vi "Main.vi"(8 "error in (no error)":errorcluster) -> (0 "error out":errorcluster)   [LabVIEW 2013]
doc: "Use this template to build a VI to use as a subVI."
uses:
  Instrument Module Typedefs/InstrumentStateEnum.ctl
  General TypeDefs/MeasurementType.ctl
  Instrument Module Typedefs/AbsorptionStateEnum.ctl
  General TypeDefs/FileSaveControllerEnum.ctl
  Measurement Typedefs/KineticNotifierDatatype.ctl
  Measurement Typedefs/MeasurementGFV.ctl
  General TypeDefs/ConfigurationDataTypeDef.ctl
  <vilib>/Utility/config.llb/Read Key (Double).vi
  <vilib>/Utility/config.llb/Read Key (Path).vi
  <vilib>/Utility/config.llb/Read Key (String).vi
  <vilib>/Utility/config.llb/Write Key (Path).vi
  <vilib>/Utility/config.llb/Write Key (String).vi
  <vilib>/Utility/config.llb/Write Key (Double).vi
  <instrlib>/Ocean Optics 2000 4000/Ocean Optics 2000 4000.lvlib
  <vilib>/Utility/config.llb/NI_LVConfig.lvlib
panel:
  in  "Export to Excel":bool
  in  "Open DB Button":bool
  in  "Save DB Button":bool
  out "Selected Wavelengths":dbl[](array[numeric])
  out "Read Status":string
  in  "Sample Name":string
  in  "MeasurementTabControl":T1(tab)=enum."Kinetic Measurement"
  out "Absorption Saved Results":T2(graph)
  out "Absorption @ wavelengths vs Time":T2(graph)
  out "Absorption Saved Results":T2(graph)
  out "Time to\nNext Save (s)":dbl=0.9000897407531738 caption="Elapsed Time (s)" format="%#.0f s"
  out "Save No.":i32
  out "FileSaveStateStatus":string="Stop" caption="File Recorder State"
  in  "Add Wavelength":bool
  in  "Remove Wavelength":bool
  in  "Measurement Type":T3=enum."Kinetic"
  in  "Req. No. of Saves":i32=1 min=1 max=10000 step=1
  in  "Enable\nAutomatic\nStop":bool=TRUE
  in  "Pause":bool caption="Start Cooling/Heating"
  in  "Stop Saves":bool caption="Start Cooling/Heating"
  in  "Record":bool caption="Start Cooling/Heating"
  in  "Time Between Consecutive Frames (sec)":dbl=1.0 caption="Time Between \nConsecutive \nSaves (sec)" min=0.0 max=3600.0 step=0.1 format="%.1f s"
  in  "Remarks":string
  out "Goal":string
  out "Experiment Name":string="tes"
  in  "NewExperiment":bool
  out "File Path":path=path "E:/LINKAM Measurements_Naama/20140915"
  in  "stop":bool
  in  "error in (no error) 2":errorcluster
  in  "Measurement Control":T4(tab)=enum."Setup Absorption Measurement"
  out "Selected Spectrometer":refnum<visa-resource-name>="USB650"
  in  "Save Calibration":bool
  out "Current State":T5=enum."Continuous Measurement"
  in  "Configure":bool
  in  "Continuous Measurement":bool
  in  "Stop Measurements":bool
  in  "Delay between measurements (ms)":i32=10 min=10 max=2000 format="%.0f ms"
  in  "Integration time (ms)":i32=120 min=10 max=2000 format="%.0f ms"
  in  "Light Strobe(On/Off)":bool=TRUE
  in  "Offset in Wavlength (nm)":dbl=9.0 min=0.0 max=100.0 format="%.2g nm"
  out "Spectrometer Raw Data":T6(graph)
  out "Live Spectrum":T6(graph)
  in  "Light Strobe Control":bool=TRUE
  in  "Number of\nsamples to average":i32=1 min=1 max=100 step=1
  in  "Take Ref Spectrum":bool
  out "Live Absorption Spectrum":T6(graph)
  out "Reference Spectrum":T6(graph)
  out "Dark Spectrum":T6(graph)
  in  "Take Dark Spectrum":bool
  out "Live samples for average":i32=1
  # "Experiment Data and File Recorder"
  # "File Recorder"
  # "Developed by Lior Segev\nsegev.lior@gmail.com\nYinon Rudich's Group\nDepartment of Earth and Planetary Sciences\n17 Sep 2014\nVer 1.0"
  # "Spectrometer Settings"
  # "Spectrometer Controller"
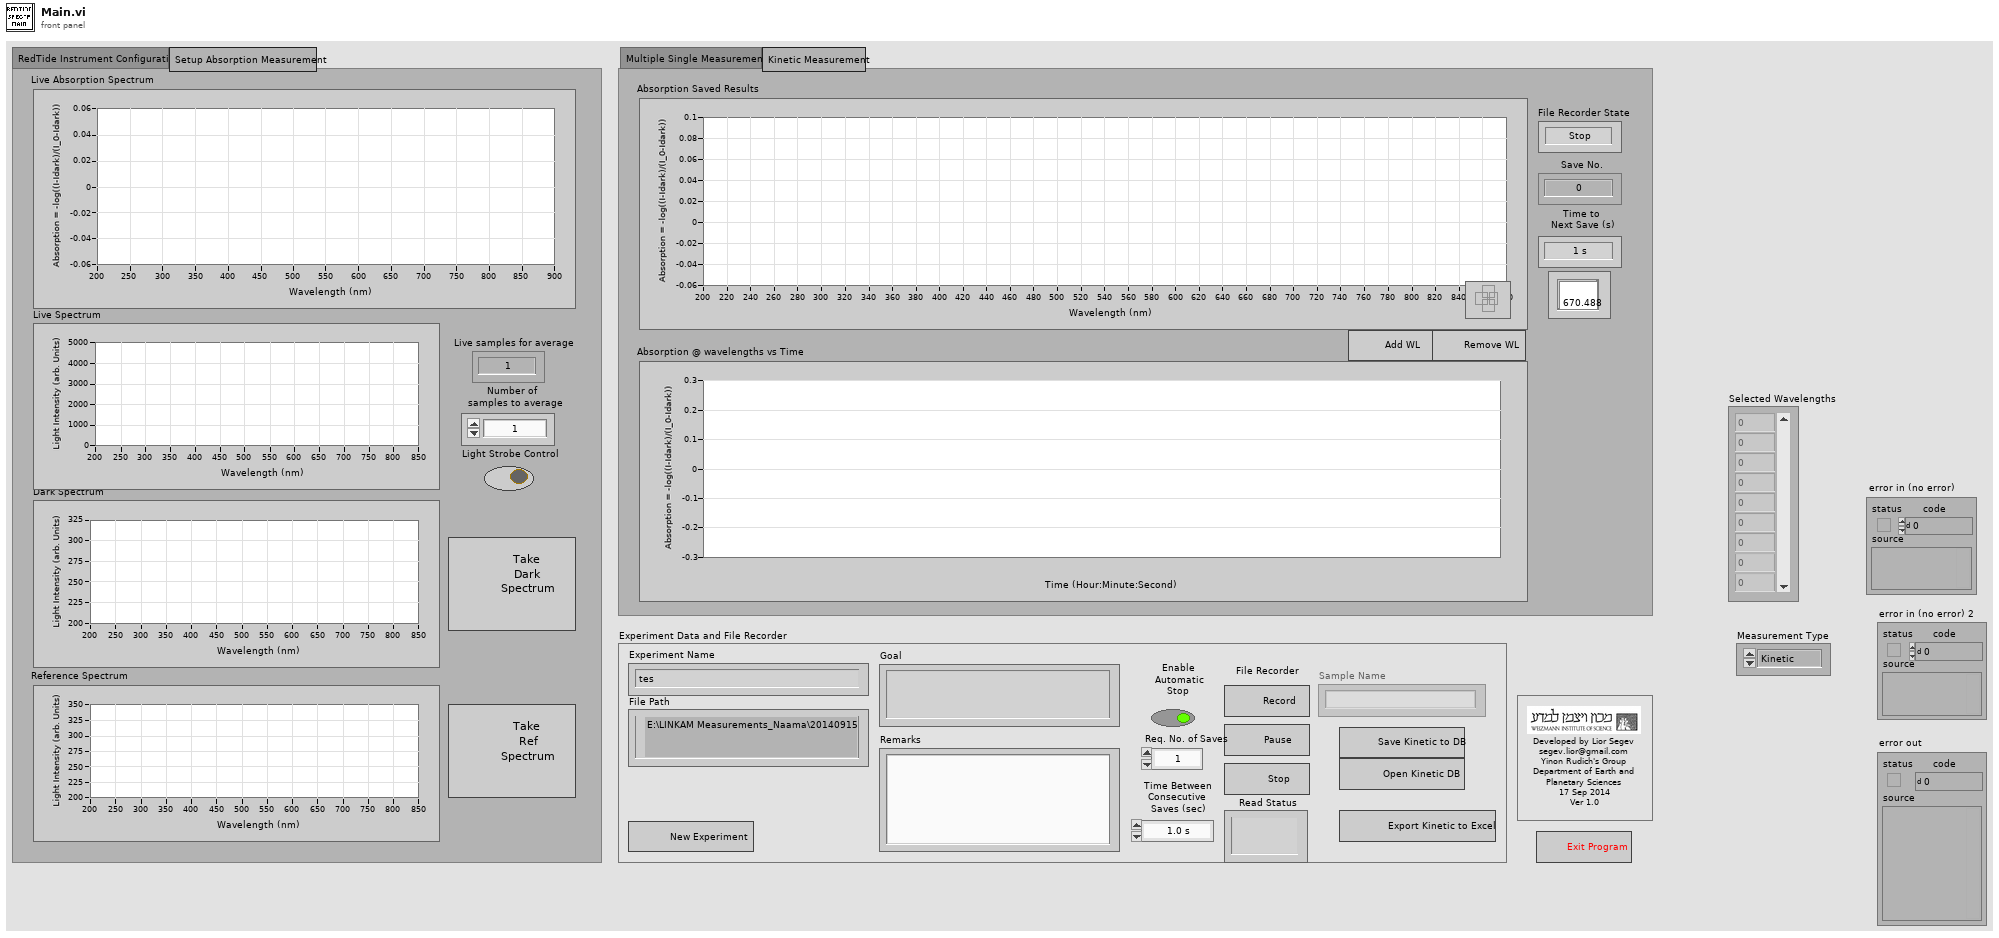
[diagram p1: front panel]
types:
  T1 = enum32{"Multiple Single Measurements", "Kinetic Measurement"}
  T2 = cluster{"Wavelength (nm)":dbl[], "Absorption":dbl[]}[]
  T3 = typedef "MeasurementType.ctl" = enum16{"Single Meas", "Kinetic"}
  T4 = enum32{"RedTide Instrument Configuration", "Setup Absorption Measurement"}
  T5 = typedef "InstrumentStateEnum.ctl" = enum16{"Error Handler", "Configure", "Stopped", "Continuous Measurement", "Single Measurement"}
  T6 = cluster{"Wavelength (nm)":dbl[], "Spectrum by Pixels":dbl[]}
  T7 = typedef "MeasurementGFV.ctl" = enum16{"Export To Excel", "GetExperimentGoalRemarks", "Load Single DB", "Save Single 2 DB", "Load Kinetic DB", "Save Kinetic 2 DB", "Get List of Wavelength", "Remove Wavelength", "Add Wavelength", "Get Sample Names", "Insert Sample Name", "Update Kinetic Display", "Update Single Display", "Init", "Insert General", "Init Single Measurement", "Insert Single Measurement", "Insert Kinetic Measurement", "Init Kinetic Measurment", "Init General"}
  T8 = enum8{"Enabled", "Disabled", "Disabled and Grayed Out"}
  T9 = typedef "KineticNotifierDatatype.ctl" = cluster{"Wavelength (nm)":dbl[], "Dark_spectrum":dbl[], "Meas_spectrum":dbl[], "Ref_spectrum":dbl[], "Absorption_spectrum":dbl[]}
  T10 = typedef "FileSaveControllerEnum.ctl" = enum16{"Record", "Pause", "Stop", "Init"}
  T11 = typedef "ConfigurationDataTypeDef.ctl" = cluster{"Experiment Name":string, "File Path":path, "Goal":string, "Remarks":string, "Time Between Consecutive Frames (sec)":dbl, "Rq. No. of saves":i32, "Enable\nAutomatic\nStop":bool, "Measurement Type":T3, "File Name":string, "Choose Spectrometer":refnum<visa-resource-name>, "Integration time (ms)":i32, "Delay between measurements (ms) ":i32, "Offset in Wavlength (nm)":dbl}
  T12 = typedef "AbsorptionStateEnum.ctl" = enum16{"RecieveMeasurement", "WaitingForMeasurements"}
  T13 = cluster{"AbsMeas":T12, "Raw Meas":cluster{"Wavelength (nm)":dbl[], "Spectrum by Pixels":dbl[]}}
  T14 = typedef "NI_LVConfig.lvlib/Config Data RefNum.ctl" = refnum<k1>
  T15 = cluster{"Absorption Saved Results":refnum<vi>, "Absorption @ wavelengths vs Time":refnum<vi>, "Selected Wavelengths":refnum<vi>}
  T16 = cluster{"AbsMeas":T12, cluster{"Wavelength (nm)":dbl[], "Spectrum by Pixels":dbl[]}}
  T17 = cluster{"Experiment Name":string, "Goal":string, "Remarks":string}
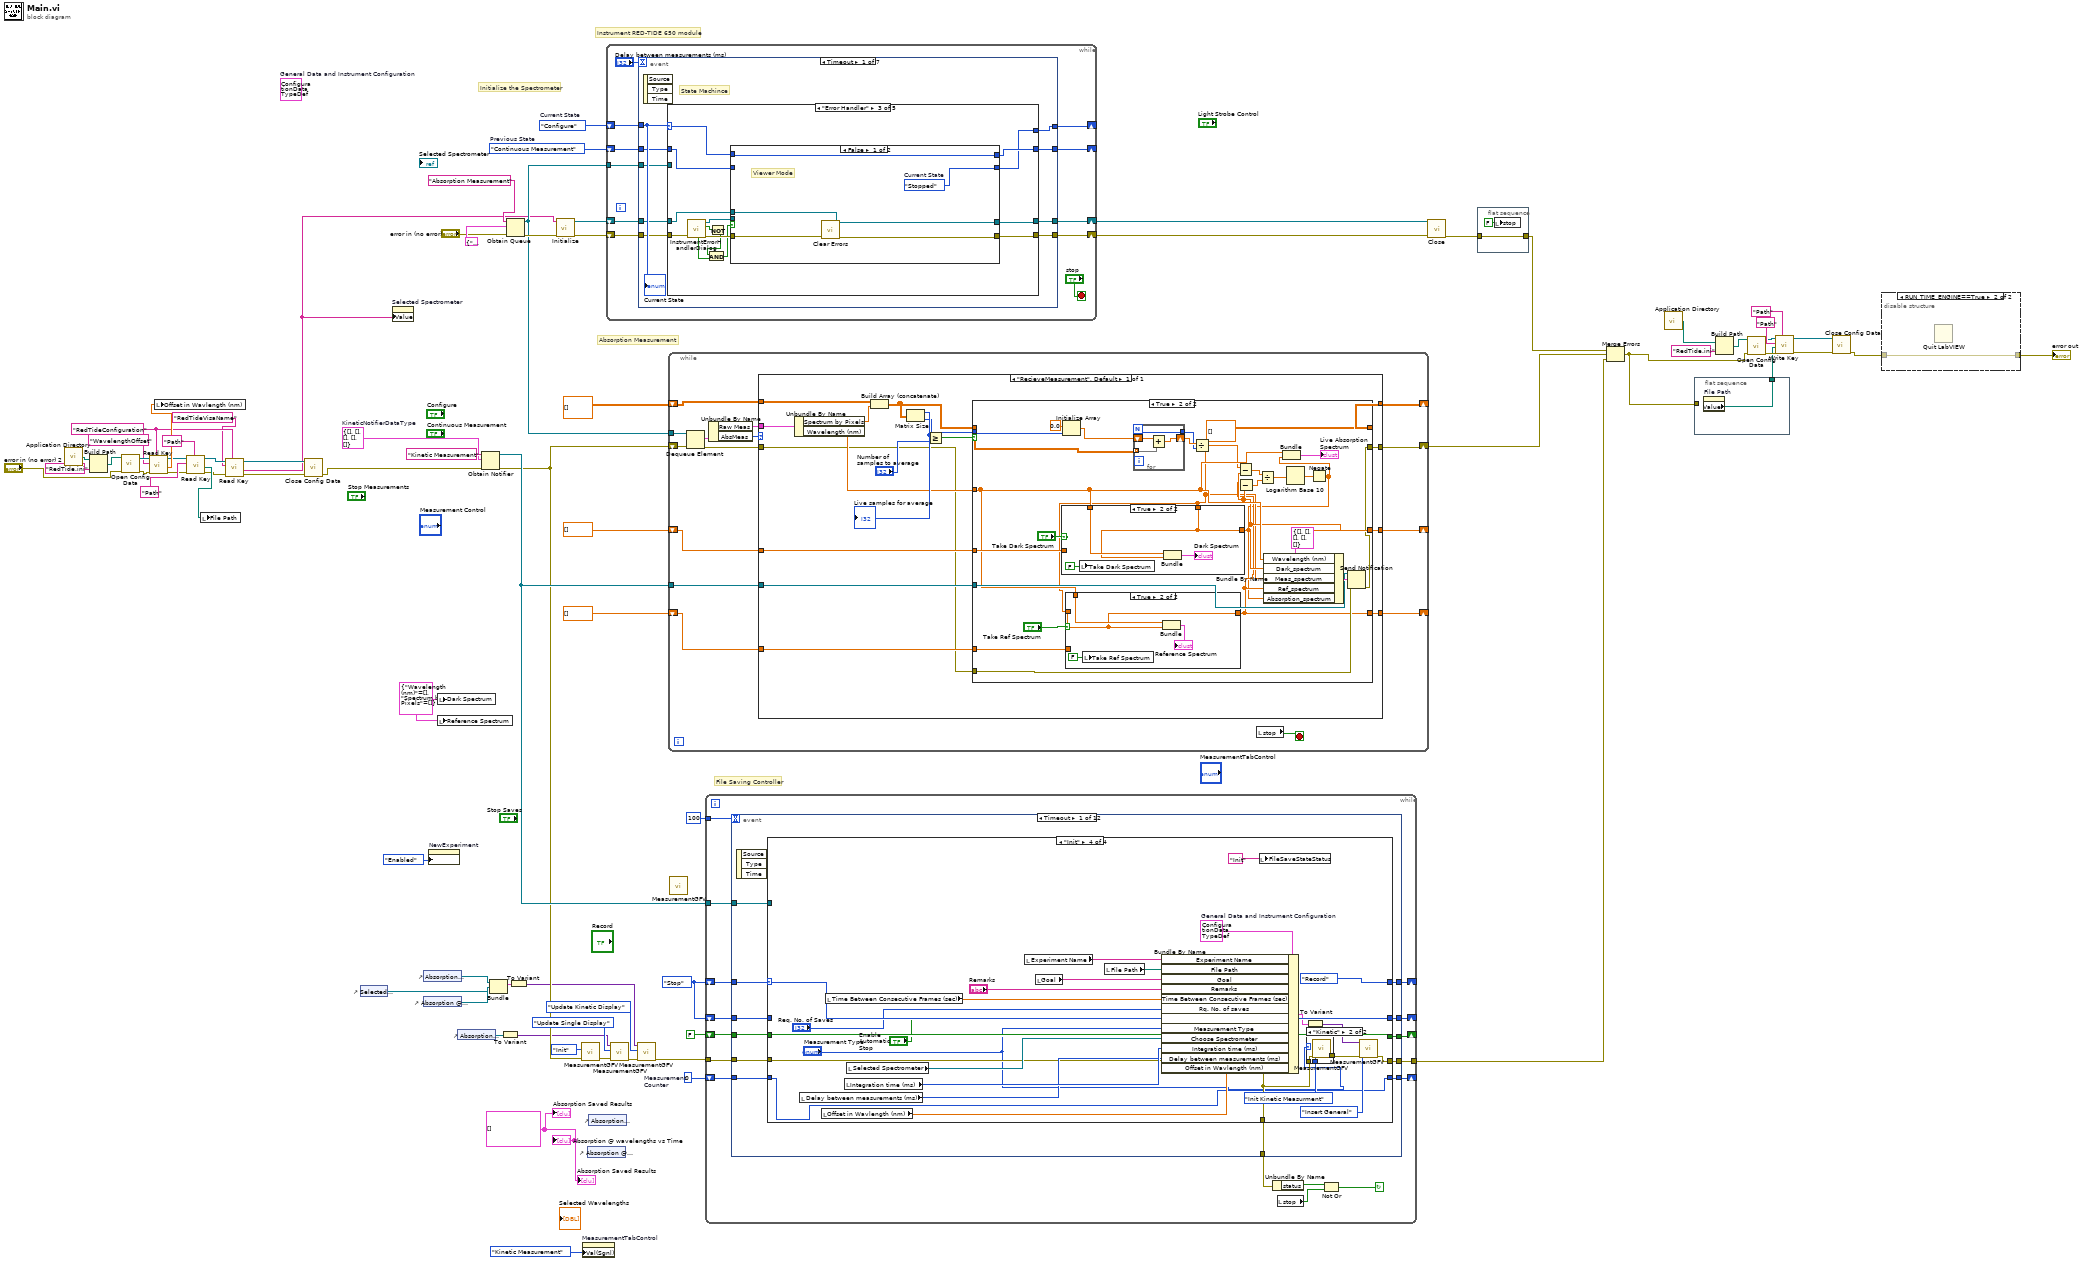
[diagram p0: block diagram]
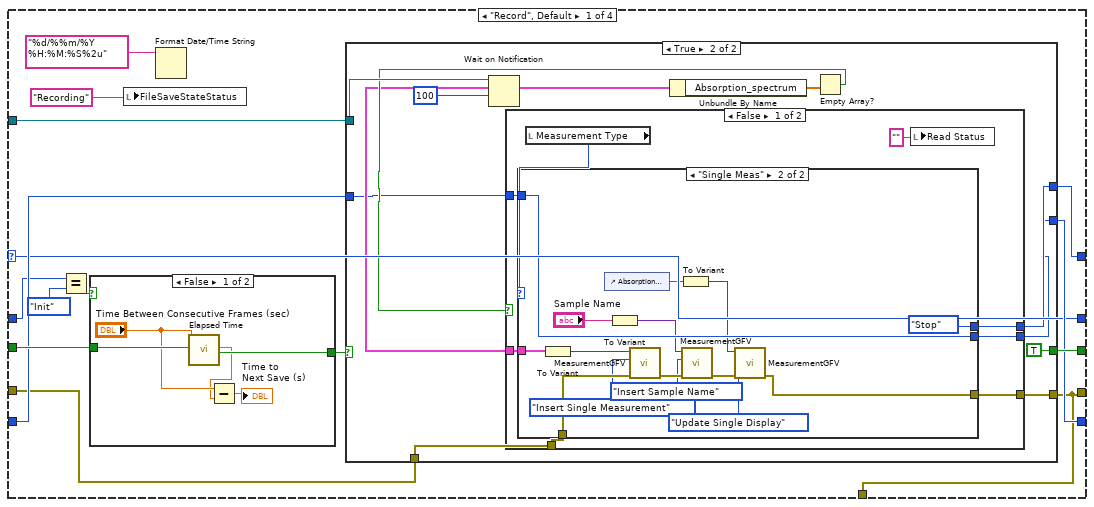
[diagram p3: hidden frame]
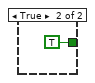
[diagram p4: hidden frame]
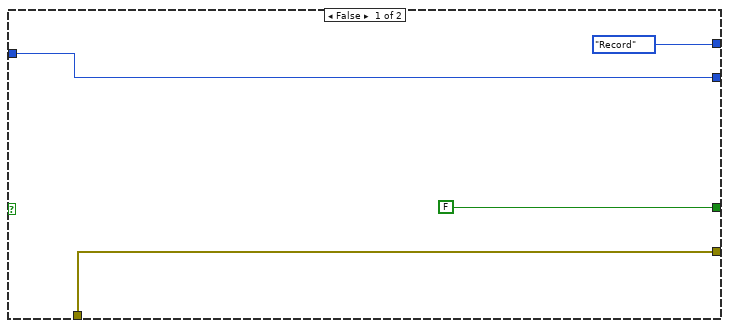
[diagram p5: hidden frame]
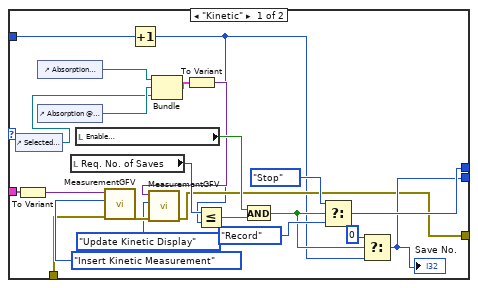
[diagram p6: hidden frame]
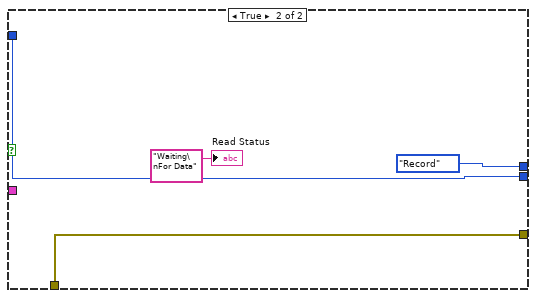
[diagram p7: hidden frame]
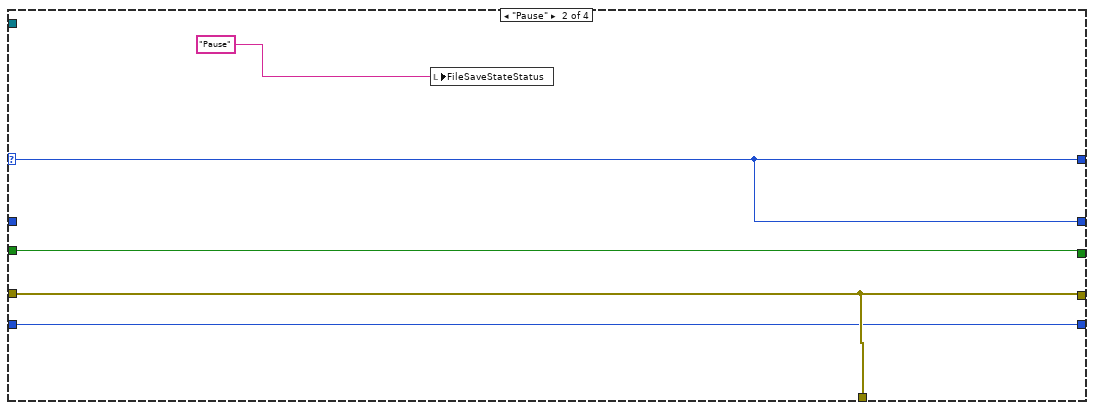
[diagram p8: hidden frame]
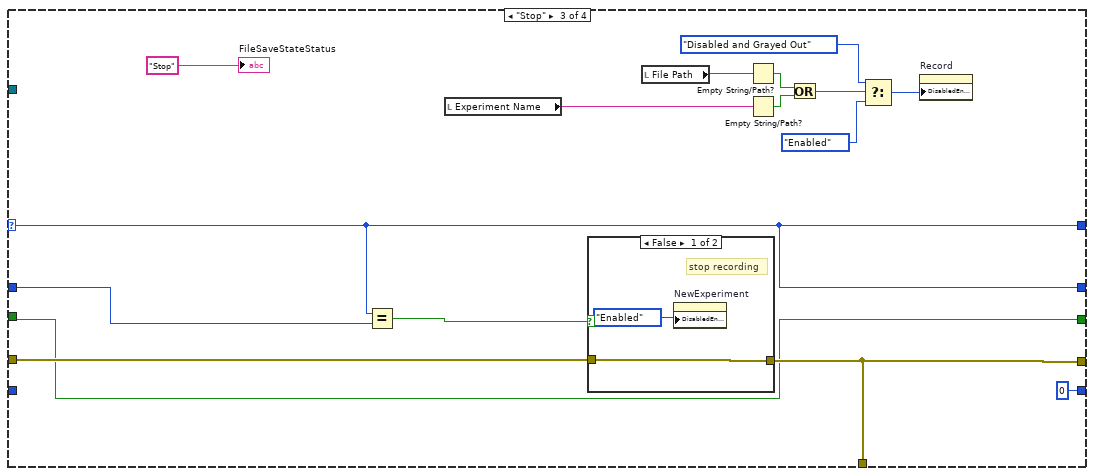
[diagram p9: hidden frame]
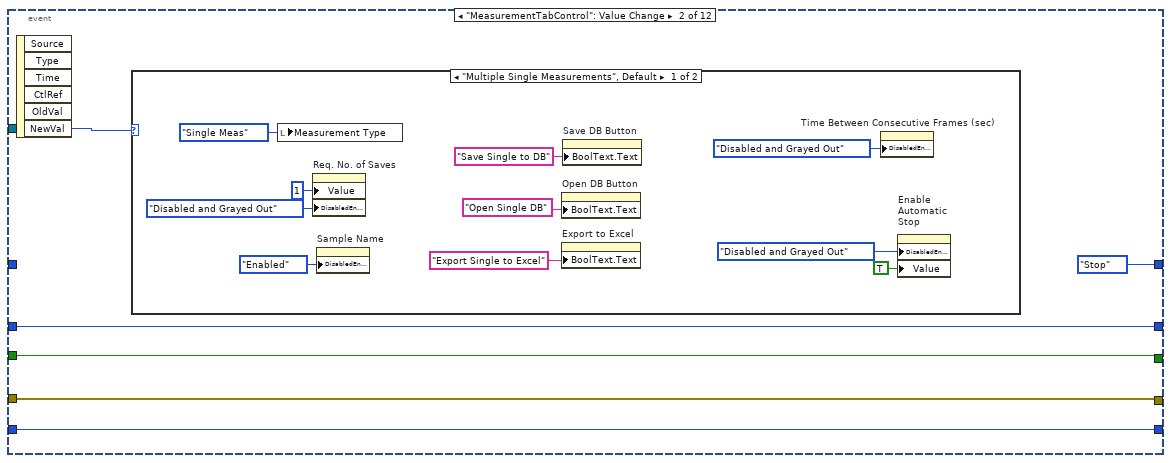
[diagram p12: hidden frame]
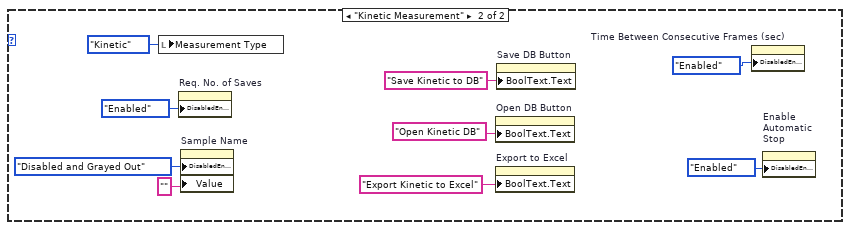
[diagram p13: hidden frame]
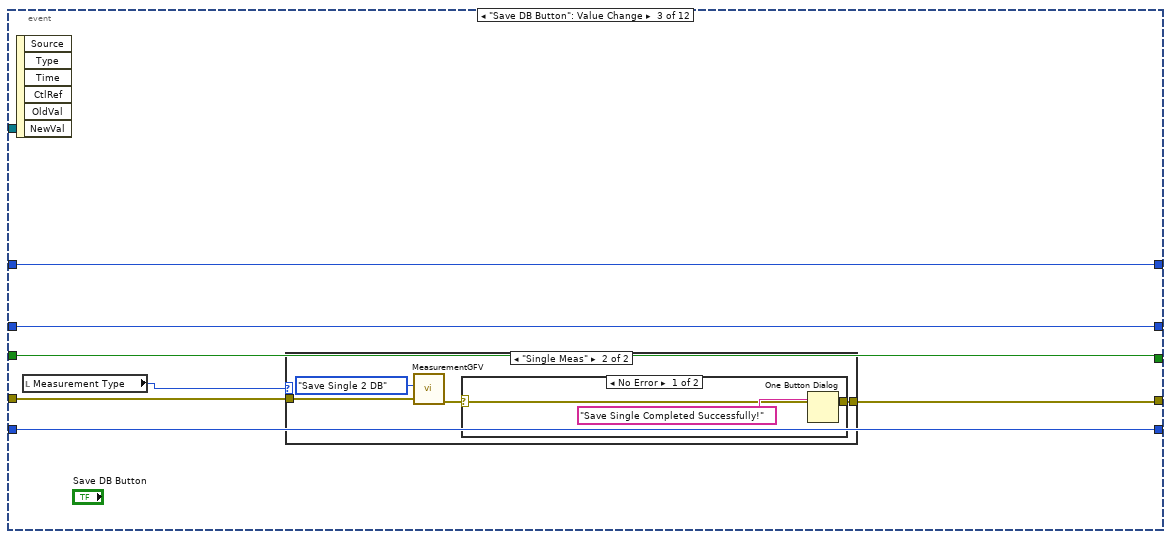
[diagram p14: hidden frame]
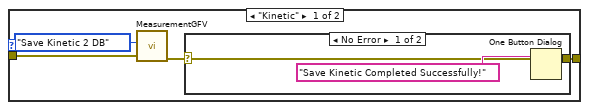
[diagram p15: hidden frame]
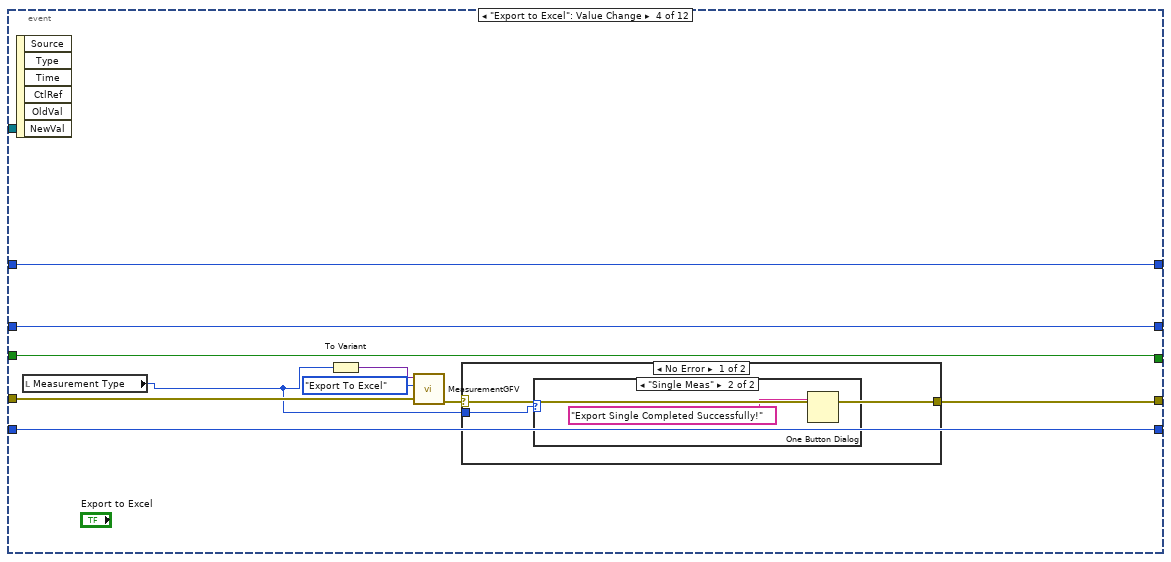
[diagram p18: hidden frame]
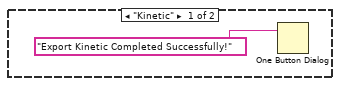
[diagram p19: hidden frame]
diagram:
  w3 = "RedTideConfiguration" ("section")
  w51 = T6 {"Wavelength (nm)"=[], "Spectrum by Pixels"=[]} ("Dark Spectrum")
  w50 = T2 []
  w52 = 0  # Measurement Counter
  w56 = T9 {"Wavelength (nm)"=[], "Dark_spectrum"=[], "Meas_spectrum"=[], "Ref_spectrum"=[], "Absorption_spectrum"=[]}  # KineticNotifierDataType
  w58 = FileSaveControllerEnum."Stop"
  (unwired) T11 {"Experiment Name"="", "File Path"=path "E:/LINKAM Measurements_Naama", "Goal"="", "Remarks"="", "Time Between Consecutive Frames (sec)"=1.0, "Rq. No. of saves"=1, "Enable\nAutomatic\nStop"=TRUE, "Measurement Type"=enum."Single Meas", "File Name"="", "Choose Spectrometer"="USB650", "Integration time (ms)"=100, "Delay between measurements (ms) "=10, "Offset in Wavlength (nm)"=9.0}  # General Data and Instrument Configuration
  w72 = InstrumentStateEnum."Continuous Measurement"  # Previous State
  w74 = InstrumentStateEnum."Configure"  # Current State
  # "File Saving Controller"
  # "Absorption Measurement"
  # "Initialize the Spectrometer"
  # "Instrument RED-TIDE 650 module"
  n1 = call <vilib>:"Application Directory.vi"() -> ("Application Directory"=w34:path)
  n2 = Build Path(base path=w34, name or relative path="RedTide.ini") -> (appended path=w32:path)
  n3 = call <vilib>:"Open Config Data.vi"("error in (no error)"="error in (no error) 2", "configuration file path"=w32) -> ("error out"=w29:errorcluster, "refnum"=w31:T14)  [unwired: 7 in, 1 out]
  n4 = call-poly <vilib>:"Read Key.vi"("section"=w3, "error in (no error)"=w29, "key"="WavelengthOffset", "refnum"=w31) -> ("error out"=w6:errorcluster, "value"=w28:dbl, "refnum out"=w13:T14)  [unwired: 4 in, 1 out]
  n5 = local write "Offset in Wavlength (nm)"(w28) -> ()
  n6 = call-poly <vilib>:"Read Key.vi"("section"="Path", "error in (no error)"=w6, "key"="Path", "refnum"=w13) -> ("error out"=w5:errorcluster, "value"=w10:path, "refnum out"=w8:T14)  [unwired: 4 in, 1 out]
  n7 = local write "File Path"(w10) -> ()
  n8 = call-poly <vilib>:"Read Key.vi"("section"=w3, "error in (no error)"=w5, "key"="RedTideVisaName" ("section"), "refnum"=w8) -> ("error out"=w4:errorcluster, "value"=w1:string, "refnum out"=w7:T14)  [unwired: 4 in, 1 out]
  n9 = call <vilib>:"Close Config Data.vi"("error in (no error)"=w4, "refnum"=w7) -> ("error out"=w26:errorcluster)  [unwired: 8 in, 1 out]
  n10 = control-ref of="Selected Wavelengths"() -> (w36:refnum<vi>)
  n11 = property on="Selected Spectrometer" class="VISAName"("Value"=w1) -> ()  [unwired: 2 in, 2 out]
  n12 = control-ref of="Absorption Saved Results"() -> (w39:refnum<vi>)
  n13 = control-ref of="Absorption @ wavelengths vs Time"() -> (w38:refnum<vi>)
  n14 = property on="NewExperiment" class="Bool"("DisabledEnum"=T8."Enabled" ("Disabled")) -> ()  [unwired: 2 in, 2 out]
  n15 = local write "Dark Spectrum"(w51) -> ()
  n16 = local write "Reference Spectrum"(w51) -> ()
  n17 = control-ref of="Absorption Saved Results"() -> (w45:refnum<vi>)
  n18 = Obtain Notifier(name (unnamed)="Kinetic Measurement", notification data type=w56, error in (no error)=w26) -> (notifier out=w55:refnum<notifier>, error out=w49:errorcluster)  [unwired: 1 in, 1 out]
  n19 = Bundle("Absorption Saved Results"=w39, "Absorption @ wavelengths vs Time"=w38, "Selected Wavelengths"=w36) -> (w40:T15)  [unwired: 1 in]
  n20 = To Variant(anything=w45) -> (Variant=w44:variant)
  n21 = Obtain Queue(name (unnamed)="Absorption Measurement", element data type=T13 {"AbsMeas"=enum."WaitingForMeasurements", "Raw Meas"={"Wavelength (nm)"=[], "Spectrum by Pixels"=[]}}, error in (no error)="error in (no error)") -> (queue out=w66:refnum<queue>, error out=w68:errorcluster)  [unwired: 2 in, 1 out]
  n22 = To Variant(anything=w40) -> (Variant=w37:variant)
  n23 = call <instrlib>:"Initialize.vi"("error in (no error)"=w68, "VISA resource name"=w1) -> ("error out"=w76:errorcluster, "VISA resource name out"=w77:refnum<visa-resource-name>)  [unwired: 8 in]
  n24 = call "MeasurementGFV.vi"("error in (no error)"=w49, "MeasuremetnGFVEnum"=MeasurementGFV."Init") -> ("error out"=w47:errorcluster)  [unwired: 8 in, 1 out]
  n25 = property on="MeasurementTabControl" class="TabCtl (strict)"("Val(Sgnl)"=T1."Kinetic Measurement" ("MeasurementTabControl")) -> ()  [unwired: 2 in, 2 out]
  n26 = control-ref of="Absorption @ wavelengths vs Time"() -> ()  [unwired: 1 out]
  n27 = control-ref of="Absorption Saved Results"() -> ()  [unwired: 1 out]
  n28 = while {
    shift-right: [w84] -> w75
    shift-left: w76 -> [w85]
    shift-right: [w80] -> _
    shift-left: w74 -> [w87]
    shift-right: [w79] -> _
    shift-left: w72 -> [w82]
    shift-right: [w83] -> w73
    shift-left: w77 -> [w86]
    tunnel: w66 -> [w78]
    stop <- "stop" stop-if-true
    n29 = event shown="[0] Timeout" {
      selector: _ -> [_ _ _ _ _ _ _]
      dyn-events: _ -> [_ _ _ _ _ _ _]
      timeout: "Delay between measurements (ms)" -> [_ _ _ _ _ _ _]
      tunnel: w87 -> [w97 w192 w209 _ _ _ _]
      tunnel: w86 -> [w96 w195 w211 w216 w220 w224 w230]
      tunnel: w85 -> [w95 w194 w199 w215 w219 w223 w229]
      tunnel: [w94 w194 w198 w215 w219 w223 w229] -> w84
      tunnel: [w93 w195 w211 w216 w220 w224 w230] -> w83
      tunnel: w82 -> [w92 w193 w210 w214 w218 w222 w227]
      tunnel: [w90 w192 w209 InstrumentStateEnum."Configure" ("Previous State") InstrumentStateEnum."Stopped" ("Previous State") InstrumentStateEnum."Continuous Measurement" ("Previous State") InstrumentStateEnum."Configure" ("Previous State")] -> w80
      tunnel: [w91 w193 w210 w214 w218 w222 w227] -> w79
      tunnel: w78 -> [w89 _ _ _ _ _ _]
      event Timeout {
        # "State Machince"
        n30 = event-data() -> ()  [unwired: 1 in, 3 out]
        n31 = case shown="\"Error Handler\"" w97 {
          selector: w97 -> [w103 w112 w118 w158 w183]
          tunnel: w96 -> [w107 w113 w123 w174 w191]
          tunnel: w95 -> [w106 w114 w128 w173 w190]
          tunnel: [w104 w114 w126 w159 w187] -> w94
          tunnel: [w105 w113 w125 w170 w186] -> w93
          tunnel: w92 -> [w99 _ w117 _ _]
          tunnel: [w103 w112 w116 w156 w183] -> w91
          tunnel: [w98 w112 w115 w157 InstrumentStateEnum."Stopped"] -> w90
          tunnel: w89 -> [_ _ _ w165 _]
          frame "Configure" {
            n32 = call <instrlib>:"Configure Integration Time.vi"("error in (no error)"=w106, "Integration Time (6000)"="Integration time (ms)", "VISA resource name"=w107) -> ("error out"=w109:errorcluster, "VISA resource name out"=w110:refnum<visa-resource-name>)  [unwired: 7 in]
            n33 = call <instrlib>:"Configure Strobe.vi"("error in (no error)"=w109, "Enable Strobe (Disabled)"="Light Strobe(On/Off)", "VISA resource name"=w110) -> ("error out"=w104:errorcluster, "VISA resource name out"=w105:refnum<visa-resource-name>)  [unwired: 7 in]
            n34 = Equal?(x=w99, y=InstrumentStateEnum."Configure" ("Previous State")) -> (x = y?=w101:bool)
            n35 = Select(t=InstrumentStateEnum."Continuous Measurement" ("Previous State"), s=w101, f=w99) -> (s? t:f=w98:T5)
          }
          frame "Stopped", Default {
          }
          frame "Error Handler" {
            n36 = call "InstrumentErrorHandlerDialog.vi"("error in (no error)"=w128) -> ("error out"=w127:errorcluster, "Enter Viewer Mode Out"=w122:bool, "Spectrometer Out"=w124:refnum<visa-resource-name>, "Add Entry Pressed?"=w120:bool)  [unwired: 7 in]
            n37 = Not(x=w122) -> (.not. x?=w121:bool)
            n38 = And(x=w121, y=w120) -> (x .and. y?=w119:bool)
            n39 = case shown="False" w119 {
              tunnel: w127 -> [w130 w141]
              tunnel: [w129 w138] -> w126
              tunnel: w124 -> [_ w140]
              tunnel: [w133 w136] -> w125
              tunnel: w123 -> [w133 _]
              tunnel: w118 -> [w131 w135]
              tunnel: w117 -> [_ w134]
              tunnel: [w131 w135] -> w116
              tunnel: [w132 w134] -> w115
              frame False {
                w132 = InstrumentStateEnum."Stopped"  # Current State
                # "Viewer Mode"
                n40 = call <vilib>:"Clear Errors.vi"("error in (no error)"=w130) -> ("error out"=w129:errorcluster)  [unwired: 6 in]
              }
              frame True {
                n41 = local write "Selected Spectrometer"(w140) -> ()
                n42 = call <instrlib>:"Initialize.vi"("error in (no error)"=w141, "VISA resource name"=w140) -> ("error out"=w139:errorcluster, "VISA resource name out"=w137:refnum<visa-resource-name>)  [unwired: 8 in]
                n43 = case shown="No Error" w139 {
                  selector: w139 -> [w150 w155]
                  tunnel: [w148 w155] -> w138
                  tunnel: w137 -> [w142 w154]
                  tunnel: [w142 w154] -> w136
                  frame No Error {
                    n44 = call <vilib>:"Application Directory.vi"() -> ("Application Directory"=w151:path)
                    n45 = Build Path(base path=w151, name or relative path="RedTide.ini") -> (appended path=w153:path)
                    n46 = call <vilib>:"Open Config Data.vi"("error in (no error)"=w150, "configuration file path"=w153) -> ("error out"=w146:errorcluster, "refnum"=w147:T14)  [unwired: 7 in, 1 out]
                    n47 = call-poly <vilib>:"Write Key.vi"("section"="RedTideConfiguration", "error in (no error)"=w146, "value"=w142, "key"="RedTideVisaName" ("section"), "refnum"=w147) -> ("error out"=w149:errorcluster, "refnum out"=w143:T14)  [unwired: 4 in, 1 out]
                    n48 = call <vilib>:"Close Config Data.vi"("error in (no error)"=w149, "refnum"=w143) -> ("error out"=w148:errorcluster)  [unwired: 8 in, 1 out]
                  }
                  frame Error {
                  }
                }
              }
            }
          }
          frame "Continuous Measurement" {
            n49 = call <instrlib>:"Read Optical Spectrum.vi"("error in (no error)"=w173, "VISA resource name"=w174) -> ("error out"=w171:errorcluster, "Spectrum by Pixels"=w168:dbl[], "VISA resource name out"=w172:refnum<visa-resource-name>)  [unwired: 6 in, 1 out]
            n50 = Array Size(array=w168) -> (size(s)=w167:i32)
            n51 = call <instrlib>:"Calculate Wavelength.vi"("error in (no error)"=w171, "Offset in Wavlength (nm)"="Offset in Wavlength (nm)", "Number of Pixels (3648)"=w167, "VISA resource name"=w172) -> ("error out"=w166:errorcluster, "Wavelength (nm)"=w169:dbl[], "VISA resource name out"=w170:refnum<visa-resource-name>)  [unwired: 5 in]
            n52 = Bundle("Wavelength (nm)"=w169, "Spectrum by Pixels"=w168) -> (w161:T6)  [unwired: 1 in]
            "Spectrometer Raw Data" <- w161
            "Live Spectrum" <- w161
            n53 = Bundle("AbsMeas"=AbsorptionStateEnum."RecieveMeasurement", w161) -> (w163:T16)  [unwired: 1 in]
            n54 = Enqueue Element(queue=w165, element=w163, error in (no error)=w166) -> (error out=w160:errorcluster)  [unwired: 1 in, 2 out]
            n55 = case shown="Error" w160 {
              selector: w160 -> [w177 w178]
              tunnel: [w177 w178] -> w159
              tunnel: w158 -> [w175 w179]
              tunnel: w158 -> [w176 _]
              tunnel: [w175 InstrumentStateEnum."Error Handler" ("Current State")] -> w157
              tunnel: [w176 w179] -> w156
              frame No Error {
              }
              frame Error {
              }
            }
          }
          frame "Single Measurement" {
            n56 = call <instrlib>:"Read Optical Spectrum.vi"("error in (no error)"=w190, "VISA resource name"=w191) -> ("error out"=w188:errorcluster, "Spectrum by Pixels"=w184:dbl[], "VISA resource name out"=w189:refnum<visa-resource-name>)  [unwired: 6 in, 1 out]
            n57 = call <instrlib>:"Calculate Wavelength.vi"("error in (no error)"=w188, "VISA resource name"=w189) -> ("error out"=w187:errorcluster, "Wavelength (nm)"=w185:dbl[], "VISA resource name out"=w186:refnum<visa-resource-name>)  [unwired: 7 in]
            n58 = Bundle("Wavelength (nm)"=w185, "Spectrum by Pixels"=w184) -> (w182:T6)  [unwired: 1 in]
            n59 = local write "Spectrometer Raw Data"(w182) -> ()
          }
        }
        "Current State" <- w97
      }
      event "Light Strobe Control": Value Change {
        n60 = event-data() -> ("NewVal"=w196:bool)  [unwired: 1 in, 5 out]
        n61 = property on="Light Strobe(On/Off)" class="Bool (strict)"("Val(Sgnl)"=w196) -> ()  [unwired: 2 in, 2 out]
      }
      event "Save Calibration": Value Change {
        n62 = event-data() -> ()  [unwired: 1 in, 6 out]
        n63 = local read "Offset in Wavlength (nm)"() -> (w197:dbl)
        n64 = call <vilib>:"Application Directory.vi"() -> ("Application Directory"=w208:path)
        n65 = Build Path(base path=w208, name or relative path="RedTide.ini") -> (appended path=w206:path)
        n66 = call <vilib>:"Open Config Data.vi"("error in (no error)"=w199, "configuration file path"=w206) -> ("error out"=w201:errorcluster, "refnum"=w205:T14)  [unwired: 7 in, 1 out]
        n67 = call-poly <vilib>:"Write Key.vi"("section"="RedTideConfiguration", "error in (no error)"=w201, "value"=w197, "key"="WavelengthOffset", "refnum"=w205) -> ("error out"=w202:errorcluster, "refnum out"=w203:T14)  [unwired: 4 in, 1 out]
        n68 = call <vilib>:"Close Config Data.vi"("error in (no error)"=w202, "refnum"=w203) -> ("error out"=w198:errorcluster)  [unwired: 8 in, 1 out]
      }
      event "Integration time (ms)", "Delay between measurements (ms)", "Light Strobe(On/Off)": Value Change {
        n69 = event-data() -> ()  [unwired: 1 in, 6 out]
        n70 = local read "Light Strobe(On/Off)"() -> (w212:bool)
        n71 = local write "Light Strobe Control"(w212) -> ()
      }
      event "Stop Measurements": Value Change {
        n72 = event-data() -> ()  [unwired: 1 in, 6 out]
        n73 = local write "Stop Measurements"(FALSE ("Stop Measurements")) -> ()
      }
      event "Continuous Measurement": Value Change {
        n74 = event-data() -> ()  [unwired: 1 in, 6 out]
        n75 = local write "Continuous Measurement"(FALSE ("Continuous Measurement")) -> ()
      }
      event "Configure": Value Change {
        n76 = event-data() -> ()  [unwired: 1 in, 6 out]
        n77 = local write "Configure"(FALSE ("Configure")) -> ()
      }
    }
  }
  n78 = call "MeasurementGFV.vi"("error in (no error)"=w47, "MeasuremetnGFVEnum"=MeasurementGFV."Update Single Display", "Variant in"=w44) -> ("error out"=w43:errorcluster)  [unwired: 7 in, 1 out]
  n79 = call "MeasurementGFV.vi"("error in (no error)"=w43, "MeasuremetnGFVEnum"=MeasurementGFV."Update Kinetic Display", "Variant in"=w37) -> ("error out"=w42:errorcluster)  [unwired: 7 in, 1 out]
  n80 = while {
    tunnel: w66 -> [w245]
    shift-right: [w239] -> w60
    shift-left: w49 -> [w244]
    shift-right: [w238] -> _
    shift-left: dbl[][] [] -> [w237]
    shift-right: [w236] -> _
    shift-left: dbl[] [] -> [w235]
    shift-right: [w234] -> _
    shift-left: dbl[] [] -> [w233]
    tunnel: w55 -> [w232]
    stop <- w246 stop-if-true
    n81 = Dequeue Element(queue=w245, error in (no error)=w244) -> (element=w241:T13, error out=w243:errorcluster)  [unwired: 1 in, 2 out]
    n82 = Unbundle By Name(w241) -> ("Raw Meas"=w240:T6, "AbsMeas"=w242:T12)
    n83 = case shown="\"RecieveMeasurement\", Default" w242 {
      tunnel: w243 -> [w248]
      tunnel: w240 -> [w263]
      tunnel: [w247] -> w239
      tunnel: [w256] -> w238
      tunnel: w237 -> [w261]
      tunnel: [w253] -> w236
      tunnel: w235 -> [w252]
      tunnel: [w251] -> w234
      tunnel: w233 -> [w250]
      tunnel: w232 -> [w249]
      frame "RecieveMeasurement", Default {
        n84 = Unbundle By Name(w263) -> ("Spectrum by Pixels"=w262:dbl[], "Wavelength (nm)"=w257:dbl[])
        n85 = Build Array (concatenate)(w261, w262) -> (w258:dbl[][])
        n86 = Matrix Size(0:w258) -> (1:w260:i32, 2:w255:i32)
        "Live samples for average" <- w260
        n87 = Greater Or Equal?(x=w260, y="Number of\nsamples to average") -> (x >= y?=w254:bool)
        n88 = case shown="True" w254 {
          tunnel: w258 -> [w267 w293]
          tunnel: w257 -> [_ w272]
          tunnel: [w267 dbl[][] []] -> w256
          tunnel: w255 -> [_ w287]
          tunnel: [w266 w271] -> w253
          tunnel: w252 -> [w266 w284]
          tunnel: [w265 w270] -> w251
          tunnel: w250 -> [w265 w282]
          tunnel: w249 -> [_ w275]
          tunnel: w248 -> [w264 w274]
          tunnel: [w264 w273] -> w247
          frame False {
          }
          frame True {
            n89 = Initialize Array(0.0 ("element"), w287) -> (w288:dbl[])
            n90 = for {
              N -> [w304]
              tunnel: w293 -> [w307] mode=indexing
              shift-right: [w306] -> w292
              shift-left: w288 -> [w305]
              tunnel: [w304] -> w291
              n91 = Add(x=w305, y=w307) -> (x+y=w306:dbl[])
            }
            n92 = Divide(x=w292, y=w291) -> (x/y=w269:dbl[])
            n93 = case shown="True" "Take Dark Spectrum" {
              tunnel: [w299 w301] -> w271
              tunnel: w269 -> [_ w301]
              tunnel: w284 -> [w299 _]
              tunnel: w272 -> [_ w302]
              frame False {
              }
              frame True {
                n94 = local write "Take Dark Spectrum"(FALSE ("Take Dark Spectrum")) -> ()
                n95 = Bundle("Wavelength (nm)"=w302, w301) -> (→"Dark Spectrum":cluster{"Wavelength (nm)":dbl[], dbl[]})  [unwired: 1 in]
              }
            }
            n96 = case shown="True" "Take Ref Spectrum" {
              tunnel: w272 -> [_ w298]
              tunnel: w269 -> [_ w295]
              tunnel: [w294 w295] -> w270
              tunnel: w282 -> [w294 _]
              frame False {
              }
              frame True {
                n97 = local write "Take Ref Spectrum"(FALSE ("Take Ref Spectrum")) -> ()
                n98 = Bundle("Wavelength (nm)"=w298, w295) -> (→"Reference Spectrum":cluster{"Wavelength (nm)":dbl[], dbl[]})  [unwired: 1 in]
              }
            }
            n99 = Subtract(x=w269, y=w271) -> (x-y=w280:dbl[])
            n100 = Subtract(x=w270, y=w271) -> (x-y=w279:dbl[])
            n101 = Divide(x=w280, y=w279) -> (x/y=w281:dbl[])
            n102 = Logarithm Base 10(1:w281) -> (0:w278:dbl[])
            n103 = Negate(x=w278) -> (-x=w268:dbl[])
            n104 = Bundle By Name(cluster=T9 {"Wavelength (nm)"=[], "Dark_spectrum"=[], "Meas_spectrum"=[], "Ref_spectrum"=[], "Absorption_spectrum"=[]} ("KineticNotifierDataType"), "Wavelength (nm)"=w272, "Dark_spectrum"=w271, "Meas_spectrum"=w269, "Ref_spectrum"=w270, "Absorption_spectrum"=w268) -> (w276:T9)
            n105 = Bundle("Wavelength (nm)"=w272, w268) -> (→"Live Absorption Spectrum":cluster{"Wavelength (nm)":dbl[], dbl[]})  [unwired: 1 in]
            n106 = Send Notification(notification=w276, notifier=w275, error in (no error)=w274) -> (error out=w273:errorcluster)  [unwired: 1 out]
          }
        }
      }
    }
    n107 = local read "stop"() -> (w246:bool)
  }
  n108 = call "MeasurementGFV.vi"() -> ()  [unwired: 10 in, 2 out]
  n109 = while {
    shift-right: [w315] -> _
    shift-left: w58 -> [w320]
    tunnel: 100 -> [w319]
    tunnel: w42 -> [w318]
    tunnel: [w317] -> w59
    shift-right: [w313] -> _
    shift-left: w58 -> [w314]
    tunnel: w55 -> [w312]
    shift-right: [w310] -> _
    shift-left: FALSE ("Time has Elapsed") -> [w311]
    shift-right: [w308] -> _
    shift-left: w52 -> [w309]
    stop <- w321 continue-if-true
    n110 = event shown="[0] Timeout" {
      selector: _ -> [_ _ _ _ _ _ _ _ _ _ _ _]
      dyn-events: _ -> [_ _ _ _ _ _ _ _ _ _ _ _]
      timeout: w319 -> [_ _ _ _ _ _ _ _ _ _ _ _]
      tunnel: w320 -> [w335 _ w503 w527 w539 w613 w650 w671 w685 _ w699 w717]
      tunnel: w318 -> [w334 w475 w502 w526 w538 w607 w649 w663 w682 w688 w695 w705]
      tunnel: [w333 w475 w501 w525 w537 w606 w649 w659 w676 w688 w694 w708] -> w317
      tunnel: [w332 _ _ _ _ _ _ _ _ _ _ _] -> w316
      tunnel: [w331 FileSaveControllerEnum."Stop" w503 w527 w539 w614 w651 w671 w685 FileSaveControllerEnum."Stop" w699 w717] -> w315
      tunnel: w314 -> [w330 w477 w504 w528 w540 _ _ w670 w684 w693 w703 w716]
      tunnel: [w329 w477 w504 w528 w540 w613 w650 w670 w684 w693 w703 w716] -> w313
      tunnel: w312 -> [w328 _ _ _ _ _ _ _ _ _ _ _]
      tunnel: w311 -> [w327 w480 w506 w530 w542 w604 w646 w673 w687 w690 w701 w711]
      tunnel: [w326 w480 w506 w530 w542 w604 w646 w673 w687 w690 w701 w711] -> w310
      tunnel: w309 -> [w325 w479 w505 w529 w541 w603 w645 w672 w686 w689 w700 w710]
      tunnel: [w324 w479 w505 w529 w541 w603 w645 w672 w686 w689 w700 w710] -> w308
      event Timeout {
        n111 = event-data() -> ()  [unwired: 1 in, 3 out]
        n112 = case shown="\"Init\"" w335 {
          selector: w335 -> [w336 w425 w441 w470]
          tunnel: [w340 w426 w429 w453] -> w333
          tunnel: w334 -> [w341 w426 w442 w456]
          tunnel: [w340 w426 w429 w456] -> w332
          tunnel: [w343 w425 w441 FileSaveControllerEnum."Record"] -> w331
          tunnel: w330 -> [w337 _ w440 _]
          tunnel: [w336 w425 w441 w470] -> w329
          tunnel: w328 -> [w347 _ _ _]
          tunnel: w327 -> [w346 w423 w428 w467]
          tunnel: [w345 w423 w428 w467] -> w326
          tunnel: w325 -> [w344 w422 _ w449]
          tunnel: [w342 w422 0 ("Measurement\nCounter") w449] -> w324
          frame "Record", Default {
            n113 = Equal?(x=w337, y=FileSaveControllerEnum."Init") -> (x = y?=w338:bool)
            n114 = case shown="False" w338 {
              tunnel: [w355 TRUE ("Time has Elapsed")] -> w348
              tunnel: w346 -> [w354 _]
              frame False {
                n115 = call "Elapsed Time"("Time Target (s)"="Time Between Consecutive Frames (sec)", "Reset"=w354) -> ("Elapsed Time (s)"=w352:dbl, "Time has Elapsed"=w355:bool)  [unwired: 10 in, 6 out]
                n116 = Subtract(x="Time Between Consecutive Frames (sec)", y=w352) -> (x-y=→"Time to\nNext Save (s)":dbl)
              }
              frame True {
              }
            }
            n117 = local write "FileSaveStateStatus"("Recording" ("Recorder Status")) -> ()
            n118 = Format Date/Time String(time format string (%c)="%d/%%m/%Y %H:%M:%S%2u") -> ()  [unwired: 2 in, 1 out]
            n119 = case shown="True" w348 {
              tunnel: w347 -> [_ w370]
              tunnel: [FALSE ("Time has Elapsed") TRUE ("Time has Elapsed")] -> w345
              tunnel: w344 -> [w359 w365]
              tunnel: [FileSaveControllerEnum."Record" w364] -> w343
              tunnel: [w359 w363] -> w342
              tunnel: w341 -> [w357 w362]
              tunnel: [w357 w361] -> w340
              frame False {
              }
              frame True {
                n120 = Wait on Notification(notifier=w370, timeout in ms (-1)=100) -> (notification=w366:T9)  [unwired: 2 in, 3 out]
                n121 = Unbundle By Name(w366) -> ("Absorption_spectrum"=w368:dbl[])
                n122 = Empty Array?(array=w368) -> (empty?=w367:bool)
                n123 = case shown="False" w367 {
                  tunnel: w366 -> [w376 _]
                  tunnel: w365 -> [w373 w419]
                  tunnel: [w378 FileSaveControllerEnum."Record"] -> w364
                  tunnel: [w377 w419] -> w363
                  tunnel: w362 -> [w375 w418]
                  tunnel: [w374 w418] -> w361
                  frame False {
                    n124 = local read "Measurement Type"() -> (w372:T3)
                    n125 = case shown="\"Single Meas\"" w372 {
                      tunnel: [w396 FileSaveControllerEnum."Stop"] -> w378
                      tunnel: [w395 w417] -> w377
                      tunnel: w376 -> [w393 w414]
                      tunnel: w375 -> [w390 w413]
                      tunnel: [w388 w403] -> w374
                      tunnel: w373 -> [w382 w417]
                      frame "Kinetic" {
                        n126 = control-ref of="Selected Wavelengths"() -> (w380:refnum<vi>)
                        n127 = To Variant(anything=w393) -> (Variant=w392:variant)
                        n128 = control-ref of="Absorption Saved Results"() -> (w386:refnum<vi>)
                        n129 = control-ref of="Absorption @ wavelengths vs Time"() -> (w387:refnum<vi>)
                        n130 = local read "Req. No. of Saves"() -> (w397:i32)
                        n131 = local read "Enable\nAutomatic\nStop"() -> (w398:bool)
                        n132 = call "MeasurementGFV.vi"("error in (no error)"=w390, "MeasuremetnGFVEnum"=MeasurementGFV."Insert Kinetic Measurement", "Variant in"=w392) -> ("error out"=w389:errorcluster)  [unwired: 7 in, 1 out]
                        n133 = Increment(x=w382) -> (x+1=w381:i32)
                        n134 = Bundle("Absorption Saved Results"=w386, "Absorption @ wavelengths vs Time"=w387, "Selected Wavelengths"=w380) -> (w384:T15)  [unwired: 1 in]
                        n135 = To Variant(anything=w384) -> (Variant=w385:variant)
                        n136 = call "MeasurementGFV.vi"("error in (no error)"=w389, "MeasuremetnGFVEnum"=MeasurementGFV."Update Kinetic Display", "Variant in"=w385) -> ("error out"=w388:errorcluster)  [unwired: 7 in, 1 out]
                        n137 = Less Or Equal?(x=w397, y=w381) -> (x <= y?=w401:bool)
                        n138 = And(x=w398, y=w401) -> (x .and. y?=w394:bool)
                        n139 = Select(t=FileSaveControllerEnum."Stop", s=w394, f=FileSaveControllerEnum."Record") -> (s? t:f=w396:T10)
                        n140 = Select(t=0 ("Measurement\nCounter"), s=w394, f=w381) -> (s? t:f=w395:i32)
                        "Save No." <- w395
                      }
                      frame "Single Meas" {
                        n141 = To Variant(anything=w414) -> (Variant=w415:variant)
                        n142 = control-ref of="Absorption Saved Results"() -> (w410:refnum<vi>)
                        n143 = To Variant(anything="Sample Name") -> (Variant=w405:variant)
                        n144 = call "MeasurementGFV.vi"("error in (no error)"=w413, "MeasuremetnGFVEnum"=MeasurementGFV."Insert Single Measurement", "Variant in"=w415) -> ("error out"=w407:errorcluster)  [unwired: 7 in, 1 out]
                        n145 = To Variant(anything=w410) -> (Variant=w409:variant)
                        n146 = call "MeasurementGFV.vi"("error in (no error)"=w407, "MeasuremetnGFVEnum"=MeasurementGFV."Insert Sample Name", "Variant in"=w405) -> ("error out"=w406:errorcluster)  [unwired: 7 in, 1 out]
                        n147 = call "MeasurementGFV.vi"("error in (no error)"=w406, "MeasuremetnGFVEnum"=MeasurementGFV."Update Single Display", "Variant in"=w409) -> ("error out"=w403:errorcluster)  [unwired: 7 in, 1 out]
                      }
                    }
                    n148 = local write "Read Status"("" ("String")) -> ()
                  }
                  frame True {
                    "Read Status" <- "Waiting\nFor Data" ("String")
                  }
                }
              }
            }
          }
          frame "Pause" {
            n149 = local write "FileSaveStateStatus"("Pause" ("Recorder Status")) -> ()
          }
          frame "Stop" {
            n150 = Equal?(x=w441, y=w440) -> (x = y?=w439:bool)
            n151 = local read "Experiment Name"() -> (w437:string)
            n152 = case shown="False" w439 {
              tunnel: w442 -> [w444 w445]
              tunnel: [w444 w445] -> w429
              frame False {
                # "stop recording"
                n153 = property on="NewExperiment" class="Bool"("DisabledEnum"=T8."Enabled" ("Disabled")) -> ()  [unwired: 2 in, 2 out]
              }
              frame True {
              }
            }
            n154 = local read "File Path"() -> (w438:path)
            n155 = Empty String/Path?(string/path=w438) -> (empty?=w435:bool)
            n156 = Empty String/Path?(string/path=w437) -> (empty?=w436:bool)
            n157 = Or(x=w435, y=w436) -> (x .or. y?=w434:bool)
            n158 = Select(t=T8."Disabled and Grayed Out" ("Disabled"), s=w434, f=T8."Enabled" ("Disabled")) -> (s? t:f=w430:T8)
            n159 = property on="Record" class="Bool (strict)"("DisabledEnum"=w430) -> ()  [unwired: 2 in, 2 out]
            "FileSaveStateStatus" <- "Stop" ("Recorder Status")
          }
          frame "Init" {
            w466 = T11 {"Experiment Name"="", "File Path"=path "E:/LINKAM Measurements_Naama", "Goal"="", "Remarks"="", "Time Between Consecutive Frames (sec)"=1.0, "Rq. No. of saves"=1, "Enable\nAutomatic\nStop"=TRUE, "Measurement Type"=enum."Single Meas", "File Name"="", "Choose Spectrometer"="USB650", "Integration time (ms)"=100, "Delay between measurements (ms) "=10, "Offset in Wavlength (nm)"=9.0}  # General Data and Instrument Configuration
            n160 = local read "Delay between measurements (ms)"() -> (w458:i32)
            n161 = local read "Offset in Wavlength (nm)"() -> (w457:dbl)
            n162 = local read "Time Between Consecutive Frames (sec)"() -> (w463:dbl)
            n163 = local read "Integration time (ms)"() -> (w459:i32)
            n164 = local read "Selected Spectrometer"() -> (w460:refnum<visa-resource-name>)
            n165 = local read "Experiment Name"() -> (w446:string)
            n166 = local read "Goal"() -> (w465:string)
            n167 = local read "File Path"() -> (w447:path)
            n168 = Bundle By Name(cluster=w466, "Experiment Name"=w446, "File Path"=w447, "Goal"=w465, "Remarks"="Remarks", "Time Between Consecutive Frames (sec)"=w463, "Rq. No. of saves"="Req. No. of Saves", "Enable\nAutomatic\nStop"="Enable\nAutomatic\nStop", "Measurement Type"="Measurement Type", "Choose Spectrometer"=w460, "Integration time (ms)"=w459, "Delay between measurements (ms)"=w458, "Offset in Wavlength (nm)"=w457) -> (w451:T11)
            n169 = local write "FileSaveStateStatus"("Init" ("Recorder Status")) -> ()
            n170 = case shown="\"Kinetic\"" "Measurement Type" {
              tunnel: w456 -> [w471 w474]
              tunnel: MeasurementGFV."Init Kinetic Measurment" ("MeasuremetnGFVEnum") -> [_ w473]
              tunnel: [w471 w472] -> w454
              frame "Single Meas", Default {
              }
              frame "Kinetic" {
                n171 = call "MeasurementGFV.vi"("error in (no error)"=w474, "MeasuremetnGFVEnum"=w473) -> ("error out"=w472:errorcluster)  [unwired: 8 in, 1 out]
              }
            }
            n172 = To Variant(anything=w451) -> (Variant=w450:variant)
            n173 = call "MeasurementGFV.vi"("error in (no error)"=w454, "MeasuremetnGFVEnum"=MeasurementGFV."Insert General", "Variant in"=w450) -> ("error out"=w453:errorcluster)  [unwired: 7 in, 1 out]
          }
        }
      }
      event "MeasurementTabControl": Value Change {
        n174 = event-data() -> ("NewVal"=w476:T1)  [unwired: 1 in, 5 out]
        n175 = case shown="\"Multiple Single Measurements\", Default" w476 {
          frame "Multiple Single Measurements", Default {
            n176 = local write "Measurement Type"(MeasurementType."Single Meas" ("Measurement Type")) -> ()
            n177 = property on="Req. No. of Saves" class="DigNum (strict)"("Value"=1 ("Req. No. of Saves"), "DisabledEnum"=T8."Disabled and Grayed Out" ("Disabled")) -> ()  [unwired: 2 in, 2 out]
            n178 = property on="Sample Name" class="Str"("DisabledEnum"=T8."Enabled" ("Disabled")) -> ()  [unwired: 2 in, 2 out]
            n179 = property on="Open DB Button" class="Bool"("BoolText.Text"="Open Single DB" ("Boolean Text.Text")) -> ()  [unwired: 2 in, 2 out]
            n180 = property on="Export to Excel" class="Bool"("BoolText.Text"="Export Single to Excel" ("Boolean Text.Text")) -> ()  [unwired: 2 in, 2 out]
            n181 = property on="Save DB Button" class="Bool"("BoolText.Text"="Save Single to DB" ("Boolean Text.Text")) -> ()  [unwired: 2 in, 2 out]
            n182 = property on="Time Between Consecutive Frames (sec)" class="DigNum (strict)"("DisabledEnum"=T8."Disabled and Grayed Out" ("Disabled")) -> ()  [unwired: 2 in, 2 out]
            n183 = property on="Enable\nAutomatic\nStop" class="Bool (strict)"("DisabledEnum"=T8."Disabled and Grayed Out" ("Disabled"), "Value"=TRUE ("Enable\nAutomatic\nStop")) -> ()  [unwired: 2 in, 2 out]
          }
          frame "Kinetic Measurement" {
            n184 = local write "Measurement Type"(MeasurementType."Kinetic" ("Measurement Type")) -> ()
            n185 = property on="Req. No. of Saves" class="DigNum (strict)"("DisabledEnum"=T8."Enabled" ("Disabled")) -> ()  [unwired: 2 in, 2 out]
            n186 = property on="Sample Name" class="Str"("DisabledEnum"=T8."Disabled and Grayed Out" ("Disabled"), "Value"="" ("Sample Name")) -> ()  [unwired: 2 in, 2 out]
            n187 = property on="Open DB Button" class="Bool"("BoolText.Text"="Open Kinetic DB" ("Boolean Text.Text")) -> ()  [unwired: 2 in, 2 out]
            n188 = property on="Export to Excel" class="Bool"("BoolText.Text"="Export Kinetic to Excel" ("Boolean Text.Text")) -> ()  [unwired: 2 in, 2 out]
            n189 = property on="Save DB Button" class="Bool"("BoolText.Text"="Save Kinetic to DB" ("Boolean Text.Text")) -> ()  [unwired: 2 in, 2 out]
            n190 = property on="Time Between Consecutive Frames (sec)" class="DigNum (strict)"("DisabledEnum"=T8."Enabled" ("Disabled")) -> ()  [unwired: 2 in, 2 out]
            n191 = property on="Enable\nAutomatic\nStop" class="Bool (strict)"("DisabledEnum"=T8."Enabled" ("Disabled")) -> ()  [unwired: 2 in, 2 out]
          }
        }
      }
      event "Save DB Button": Value Change {
        n192 = event-data() -> ()  [unwired: 1 in, 6 out]
        n193 = local read "Measurement Type"() -> (w500:T3)
        n194 = case shown="\"Single Meas\"" w500 {
          tunnel: w502 -> [w510 w517]
          tunnel: [w507 w514] -> w501
          frame "Kinetic" {
            n195 = call "MeasurementGFV.vi"("error in (no error)"=w510, "MeasuremetnGFVEnum"=MeasurementGFV."Save Kinetic 2 DB") -> ("error out"=w508:errorcluster)  [unwired: 8 in, 1 out]
            n196 = case shown="No Error" w508 {
              selector: w508 -> [w511 w513]
              tunnel: [w511 w513] -> w507
              frame No Error {
                n197 = One Button Dialog(message="Save Kinetic Completed Successfully!") -> ()  [unwired: 1 in, 1 out]
              }
              frame Error {
              }
            }
          }
          frame "Single Meas" {
            n198 = call "MeasurementGFV.vi"("error in (no error)"=w517, "MeasuremetnGFVEnum"=MeasurementGFV."Save Single 2 DB") -> ("error out"=w515:errorcluster)  [unwired: 8 in, 1 out]
            n199 = case shown="No Error" w515 {
              selector: w515 -> [w518 w520]
              tunnel: [w518 w520] -> w514
              frame No Error {
                n200 = One Button Dialog(message="Save Single Completed Successfully!") -> ()  [unwired: 1 in, 1 out]
              }
              frame Error {
              }
            }
          }
        }
      }
      event "Export to Excel": Value Change {
        n201 = event-data() -> ()  [unwired: 1 in, 6 out]
        n202 = local read "Measurement Type"() -> (w521:T3)
        n203 = To Variant(anything=w521) -> (Variant=w522:variant)
        n204 = call "MeasurementGFV.vi"("error in (no error)"=w526, "MeasuremetnGFVEnum"=MeasurementGFV."Export To Excel", "Variant in"=w522) -> ("error out"=w523:errorcluster)  [unwired: 7 in, 1 out]
        n205 = case shown="No Error" w523 {
          selector: w523 -> [w532 w535]
          tunnel: [w532 w535] -> w525
          tunnel: w521 -> [w531 _]
          frame No Error {
            n206 = case shown="\"Single Meas\"" w531 {
              frame "Kinetic" {
                n207 = One Button Dialog(message="Export Kinetic Completed Successfully!") -> ()  [unwired: 1 in, 1 out]
              }
              frame "Single Meas" {
                n208 = One Button Dialog(message="Export Single Completed Successfully!") -> ()  [unwired: 1 in, 1 out]
              }
            }
          }
          frame Error {
          }
        }
      }
      event "Open DB Button": Value Change {
        n209 = event-data() -> ()  [unwired: 1 in, 6 out]
        n210 = local read "Measurement Type"() -> (w536:T3)
        n211 = case shown="\"Kinetic\"" w536 {
          tunnel: w538 -> [w547 w576]
          tunnel: [w544 w573] -> w537
          frame "Kinetic" {
            n212 = call "File Dialog"("error in"=w547, "pattern (all files)"="*.kinetic", "pattern label"="Kinetic Measurement Files") -> ("selected path"=w543:path, "cancelled"=w546:bool, "error out"=w545:errorcluster)  [unwired: 9 in, 1 out]
            n213 = case shown="False" w546 {
              tunnel: w545 -> [w569 w571]
              tunnel: [w551 w571] -> w544
              tunnel: w543 -> [w568 _]
              frame False {
                n214 = control-ref of="Selected Wavelengths"() -> (w564:refnum<vi>)
                n215 = To Variant(anything=w568) -> (Variant=w567:variant)
                n216 = call "MeasurementGFV.vi"("error in (no error)"=w569, "MeasuremetnGFVEnum"=MeasurementGFV."Load Kinetic DB", "Variant in"=w567) -> ("error out"=w566:errorcluster)  [unwired: 7 in, 1 out]
                n217 = control-ref of="Absorption Saved Results"() -> (w562:refnum<vi>)
                n218 = control-ref of="Absorption @ wavelengths vs Time"() -> (w563:refnum<vi>)
                n219 = Bundle("Absorption Saved Results"=w562, "Absorption @ wavelengths vs Time"=w563, "Selected Wavelengths"=w564) -> (w561:T15)  [unwired: 1 in]
                n220 = To Variant(anything=w561) -> (Variant=w560:variant)
                n221 = call "MeasurementGFV.vi"("error in (no error)"=w566, "MeasuremetnGFVEnum"=MeasurementGFV."Update Kinetic Display", "Variant in"=w560) -> ("error out"=w552:errorcluster)  [unwired: 7 in, 1 out]
                n222 = call "MeasurementGFV.vi"("error in (no error)"=w552, "MeasuremetnGFVEnum"=MeasurementGFV."GetExperimentGoalRemarks") -> ("error out"=w557:errorcluster, "Variant Out"=w556:variant)  [unwired: 8 in]
                n223 = Variant To Data(error in=w557, type=T17 {"Experiment Name"="", "Goal"="", "Remarks"=""} ("output cluster"), Variant=w556) -> (data=w558:T17, error out=w551:errorcluster)
                n224 = Unbundle By Name(w558) -> ("Experiment Name"=w550:string, "Goal"=w554:string, "Remarks"=w553:string)
                n225 = local write "Experiment Name"(w550) -> ()
                n226 = local write "Goal"(w554) -> ()
                n227 = local write "Remarks"(w553) -> ()
              }
              frame True {
              }
            }
          }
          frame "Single Meas" {
            n228 = call "File Dialog2"("error in"=w576, "pattern (all files)"="*.Single", "pattern label"="Single Measurement Files") -> ("selected path"=w572:path, "cancelled"=w575:bool, "error out"=w574:errorcluster)  [unwired: 9 in, 1 out]
            n229 = case shown="False" w575 {
              tunnel: w574 -> [w595 w597]
              tunnel: [w582 w597] -> w573
              tunnel: w572 -> [w594 _]
              frame False {
                n230 = To Variant(anything=w594) -> (Variant=w593:variant)
                n231 = call "MeasurementGFV.vi"("error in (no error)"=w595, "MeasuremetnGFVEnum"=MeasurementGFV."Load Single DB", "Variant in"=w593) -> ("error out"=w592:errorcluster)  [unwired: 7 in, 1 out]
                n232 = control-ref of="Absorption Saved Results"() -> (w590:refnum<vi>)
                n233 = To Variant(anything=w590) -> (Variant=w589:variant)
                n234 = call "MeasurementGFV.vi"("error in (no error)"=w592, "MeasuremetnGFVEnum"=MeasurementGFV."Update Single Display", "Variant in"=w589) -> ("error out"=w588:errorcluster)  [unwired: 7 in, 1 out]
                n235 = call "MeasurementGFV.vi"("error in (no error)"=w588, "MeasuremetnGFVEnum"=MeasurementGFV."GetExperimentGoalRemarks") -> ("error out"=w586:errorcluster, "Variant Out"=w585:variant)  [unwired: 8 in]
                n236 = Variant To Data(error in=w586, type=T17 {"Experiment Name"="", "Goal"="", "Remarks"=""} ("output cluster"), Variant=w585) -> (data=w583:T17, error out=w582:errorcluster)
                n237 = Unbundle By Name(w583) -> ("Experiment Name"=w581:string, "Goal"=w580:string, "Remarks"=w579:string)
                n238 = local write "Experiment Name"(w581) -> ()
                n239 = local write "Goal"(w580) -> ()
                n240 = local write "Remarks"(w579) -> ()
              }
              frame True {
              }
            }
          }
        }
      }
      event "Record": Value Change {
        n241 = event-data() -> ()  [unwired: 1 in, 6 out]
        n242 = local read "Experiment Name"() -> (w611:string)
        n243 = local read "Measurement Type"() -> (w602:T3)
        n244 = local read "File Path"() -> (w612:path)
        n245 = Empty String/Path?(string/path=w612) -> (empty?=w609:bool)
        n246 = Empty String/Path?(string/path=w611) -> (empty?=w610:bool)
        n247 = case shown="\"Single Meas\", Default" w602 {
          tunnel: [w616 FALSE] -> w600
          frame "Single Meas", Default {
            n248 = call "MeasurementGFV.vi"("MeasuremetnGFVEnum"=MeasurementGFV."Get Sample Names") -> ("error out"=w621:errorcluster, "Variant Out"=w622:variant)  [unwired: 9 in]
            n249 = local read "Sample Name"() -> (w617:string)
            n250 = Variant To Data(error in=w621, type=string[] [], Variant=w622) -> (data=w619:string[])  [unwired: 1 out]
            n251 = for {
              tunnel: w619 -> [w632] mode=indexing
              shift-right: [w629] -> w616
              shift-left: FALSE -> [w628]
              tunnel: w617 -> [w627]
              n252 = Equal?(x=w632, y=w627) -> (x = y?=w631:bool)
              n253 = Select(t=TRUE, s=w631, f=w628) -> (s? t:f=w629:bool)
            }
            n254 = case shown="True" w616 {
              tunnel: [TRUE ("true") w625] -> w615
              frame False {
              }
              frame True {
                n255 = One Button Dialog(message="Sample name exists. Please choose a different sample name.") -> (true=w625:bool)  [unwired: 1 in]
              }
            }
            n256 = property on="Sample Name" class="Str"("Key Focus"=w615) -> ()  [unwired: 2 in, 2 out]
          }
          frame "Kinetic" {
          }
        }
        n257 = Or(x=w609, y=w610) -> (x .or. y?=w608:bool)
        n258 = Not(x=w608) -> (.not. x?=w601:bool)
        n259 = Not(x=w600) -> (.not. x?=w599:bool)
        n260 = And(x=w599, y=w601) -> (x .and. y?=w598:bool)
        n261 = case shown="True" w598 {
          tunnel: [w635 w644] -> w614
          tunnel: w613 -> [w635 w643]
          tunnel: w607 -> [w634 w641]
          tunnel: [w634 w640] -> w606
          frame False {
          }
          frame True {
            n262 = property on="NewExperiment" class="Bool"(error in=w641, "DisabledEnum"=T8."Disabled and Grayed Out" ("Disabled")) -> (error out=w640:errorcluster)  [unwired: 1 in, 1 out]
            n263 = Equal?(x=w643, y=FileSaveControllerEnum."Stop") -> (x = y?=w642:bool)
            n264 = Select(t=FileSaveControllerEnum."Init", s=w642, f=FileSaveControllerEnum."Record") -> (s? t:f=w644:T10)
          }
        }
        n265 = local write "Record"(FALSE ("Record")) -> ()
      }
      event "Pause": Value Change {
        n266 = event-data() -> ()  [unwired: 1 in, 6 out]
        n267 = Equal?(x=w650, y=FileSaveControllerEnum."Record") -> (x = y?=w652:bool)
        n268 = Select(t=FileSaveControllerEnum."Pause", s=w652, f=w650) -> (s? t:f=w651:T10)
      }
      event "Add Wavelength": Value Change {
        n269 = event-data() -> ()  [unwired: 1 in, 6 out]
        n270 = control-ref of="Absorption Saved Results"() -> (w661:refnum<vi>)
        n271 = property class="XYGraph (strict)"(reference=w661, error in=w663, "Active Cursor"=u32 0) -> (reference out=w667:refnum<vi>, error out=w665:errorcluster)
        n272 = control-ref of="Selected Wavelengths"() -> (w657:refnum<vi>)
        n273 = control-ref of="Absorption Saved Results"() -> (w655:refnum<vi>)
        n274 = control-ref of="Absorption @ wavelengths vs Time"() -> (w656:refnum<vi>)
        n275 = property class="XYGraph (strict)"(reference=w667, error in=w665) -> (error out=w662:errorcluster, "Cursor.Cursor X"=w666:dbl)  [unwired: 1 out]
        n276 = To Variant(anything=w666) -> (Variant=w664:variant)
        n277 = Bundle("Absorption Saved Results"=w655, "Absorption @ wavelengths vs Time"=w656, "Selected Wavelengths"=w657) -> (w654:T15)  [unwired: 1 in]
        n278 = call "MeasurementGFV.vi"("error in (no error)"=w662, "MeasuremetnGFVEnum"=MeasurementGFV."Add Wavelength", "Variant in"=w664) -> ("error out"=w660:errorcluster)  [unwired: 7 in, 1 out]
        n279 = To Variant(anything=w654) -> (Variant=w653:variant)
        n280 = call "MeasurementGFV.vi"("error in (no error)"=w660, "MeasuremetnGFVEnum"=MeasurementGFV."Update Kinetic Display", "Variant in"=w653) -> ("error out"=w659:errorcluster)  [unwired: 7 in, 1 out]
      }
      event "Remove Wavelength": Value Change {
        n281 = event-data() -> ()  [unwired: 1 in, 6 out]
        n282 = control-ref of="Selected Wavelengths"() -> (w681:refnum<vi>)
        n283 = control-ref of="Absorption Saved Results"() -> (w679:refnum<vi>)
        n284 = control-ref of="Absorption @ wavelengths vs Time"() -> (w680:refnum<vi>)
        n285 = Bundle("Absorption Saved Results"=w679, "Absorption @ wavelengths vs Time"=w680, "Selected Wavelengths"=w681) -> (w678:T15)  [unwired: 1 in]
        n286 = call "MeasurementGFV.vi"("error in (no error)"=w682, "MeasuremetnGFVEnum"=MeasurementGFV."Remove Wavelength") -> ("error out"=w677:errorcluster)  [unwired: 8 in, 1 out]
        n287 = To Variant(anything=w678) -> (Variant=w675:variant)
        n288 = call "MeasurementGFV.vi"("error in (no error)"=w677, "MeasuremetnGFVEnum"=MeasurementGFV."Update Kinetic Display", "Variant in"=w675) -> ("error out"=w676:errorcluster)  [unwired: 7 in, 1 out]
      }
      event "Stop Saves": Value Change {
        # "Save Ascii file with Experiments details"
        n289 = event-data() -> ()  [unwired: 1 in, 6 out]
        n290 = local write "Stop Saves"(FALSE ("Stop")) -> ()
      }
      event "Sample Name": Value Change {
        # "Save Ascii file with Experiments details"
        n291 = event-data() -> ()  [unwired: 1 in, 6 out]
        n292 = local write "Stop Saves"(FALSE ("Stop")) -> ()
        n293 = property on="Record" class="Bool (strict)"(error in=w695, "Val(Sgnl)"=TRUE ("Value (Signaling)")) -> (error out=w696:errorcluster)  [unwired: 1 in, 1 out]
        n294 = property on="Sample Name" class="Str"(error in=w696, "Key Focus"=TRUE) -> (error out=w694:errorcluster)  [unwired: 1 in, 1 out]
      }
      event "NewExperiment": Value Change {
        n295 = event-data() -> ()  [unwired: 1 in, 6 out]
        n296 = property on="File Path" class="Path"(error in=w705) -> (error out=w704:errorcluster, "Value"=w707:path)  [unwired: 1 in, 1 out]
        n297 = Strip Path(path=w707) -> (stripped path=w706:path)  [unwired: 1 out]
        n298 = call "NewExperimentDialog.vi"("error in (no error)"=w704, "File Path"=w706) -> ("error out"=w709:errorcluster, "Goal 2"=w713:string, "File Path 2"=w714:path, "Experiment Name 2"=w715:string, "Add Entry Pressed?"=w712:bool)  [unwired: 5 in]
        n299 = case shown="True" w712 {
          tunnel: w715 -> [_ w739]
          tunnel: w713 -> [_ w737]
          tunnel: w714 -> [_ w738]
          tunnel: w709 -> [w718 w724]
          tunnel: [w718 w725] -> w708
          frame False {
          }
          frame True {
            n300 = control-ref of="Absorption Saved Results"() -> (w734:refnum<vi>)
            n301 = control-ref of="Absorption @ wavelengths vs Time"() -> (w735:refnum<vi>)
            n302 = control-ref of="Absorption Saved Results"() -> (w729:refnum<vi>)
            n303 = call "MeasurementGFV.vi"("error in (no error)"=w724, "MeasuremetnGFVEnum"=MeasurementGFV."Init Single Measurement") -> ("error out"=w723:errorcluster)  [unwired: 8 in, 1 out]
            n304 = To Variant(anything=w729) -> (Variant=w730:variant)
            n305 = call "MeasurementGFV.vi"("error in (no error)"=w723, "MeasuremetnGFVEnum"=MeasurementGFV."Init Kinetic Measurment") -> ("error out"=w722:errorcluster)  [unwired: 8 in, 1 out]
            n306 = control-ref of="Selected Wavelengths"() -> (w719:refnum<vi>)
            n307 = Bundle("Absorption Saved Results"=w734, "Absorption @ wavelengths vs Time"=w735, "Selected Wavelengths"=w719) -> (w733:T15)  [unwired: 1 in]
            n308 = To Variant(anything=w733) -> (Variant=w736:variant)
            n309 = call "MeasurementGFV.vi"("error in (no error)"=w722, "MeasuremetnGFVEnum"=MeasurementGFV."Init General") -> ("error out"=w727:errorcluster)  [unwired: 8 in, 1 out]
            n310 = call "MeasurementGFV.vi"("error in (no error)"=w727, "MeasuremetnGFVEnum"=MeasurementGFV."Update Single Display", "Variant in"=w730) -> ("error out"=w731:errorcluster)  [unwired: 7 in, 1 out]
            n311 = call "MeasurementGFV.vi"("error in (no error)"=w731, "MeasuremetnGFVEnum"=MeasurementGFV."Update Kinetic Display", "Variant in"=w736) -> ("error out"=w725:errorcluster)  [unwired: 7 in, 1 out]
            "Experiment Name" <- w739
            "File Path" <- w738
            "Goal" <- w737
          }
        }
      }
    }
    n312 = Unbundle By Name(w316) -> ("status"=w322:bool)
    n313 = local read "stop"() -> (w323:bool)
    n314 = Not Or(1:w323, 2:w322) -> (0:w321:bool)
  }
  n315 = call <instrlib>:"Close.vi"("error in (no error)"=w75, "VISA resource name"=w73) -> ("error out"=w71:errorcluster)  [unwired: 9 in]
  n316 = flat-sequence {
    tunnel: w71 -> [w740]
    tunnel: [w740] -> w61
    frame #0 {
      n317 = local write "stop"(FALSE ("stop")) -> ()
    }
  }
  n318 = Merge Errors(w61, w60, w59) -> (w9:errorcluster)
  n319 = call <vilib>:"Application Directory.vi"() -> ("Application Directory"=w16:path)
  n320 = flat-sequence {
    tunnel: [w742] -> w14
    tunnel: w9 -> [_]
    frame #0 {
      n321 = property on="File Path" class="Path"() -> ("Value"=w742:path)  [unwired: 2 in, 2 out]
    }
  }
  n322 = Build Path(base path=w16, name or relative path="RedTide.ini") -> (appended path=w18:path)
  n323 = call <vilib>:"Open Config Data.vi"("error in (no error)"=w9, "configuration file path"=w18) -> ("error out"=w23:errorcluster, "refnum"=w19:T14)  [unwired: 7 in, 1 out]
  n324 = call-poly <vilib>:"Write Key.vi"("section"="Path", "error in (no error)"=w23, "value"=w14, "key"="Path", "refnum"=w19) -> ("error out"=w22:errorcluster, "refnum out"=w21:T14)  [unwired: 4 in, 1 out]
  n325 = call <vilib>:"Close Config Data.vi"("error in (no error)"=w22, "refnum"=w21) -> ("error out"=w15:errorcluster)  [unwired: 8 in, 1 out]
  n326 = disable-structure shown="RUN_TIME_ENGINE==True" {
    disable-tunnel: w15 -> [w743 w744]
    disable-tunnel: [w743 w744] -> w25
    frame condition #0 (active) {
    }
    frame condition #1 {
      n327 = Quit LabVIEW() -> ()  [unwired: 1 in]
    }
  }
  "error out" <- w25
  "Absorption @ wavelengths vs Time" <- w50
  "Absorption Saved Results" <- w50
  "Absorption Saved Results" <- w50
